vi "Plink Test.vi"() -> ()   [LabVIEW 2024]
panel:
  in  "format string":string="plink -pw changeme -batch -no-antispoof root@%s \"/opt/bin/maglab_rp_info\""
  in  "wait until completion? (T)":bool=TRUE
  in  "IP":string="192.168.1.120"
  in  "run minimized? (F)":bool
  out "return code":i32
  out "standard error":string
  out "standard output":string
  out "command":string
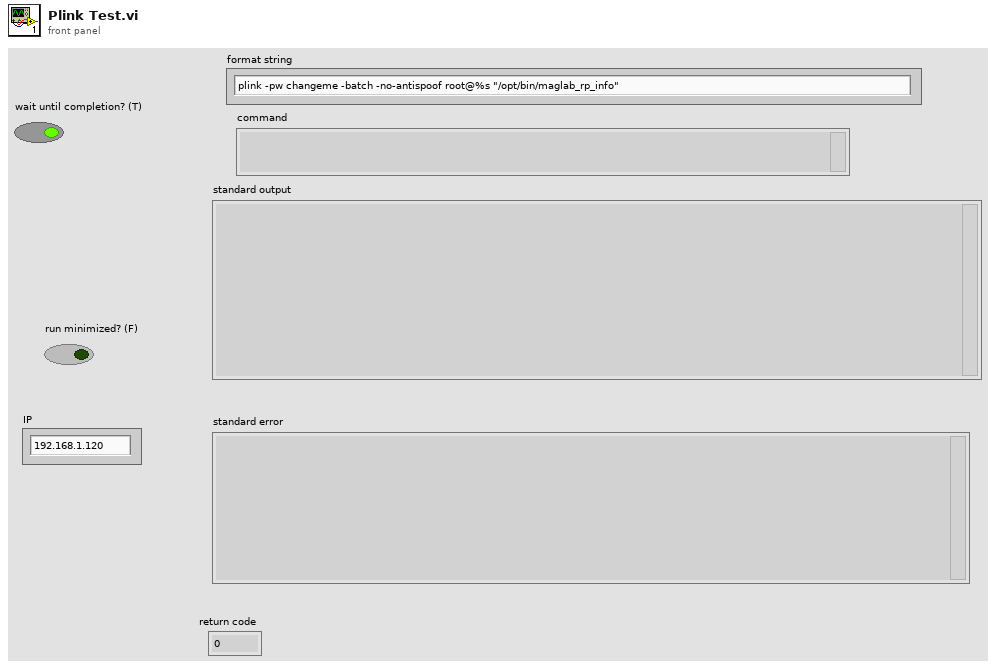
[diagram p1: front panel]
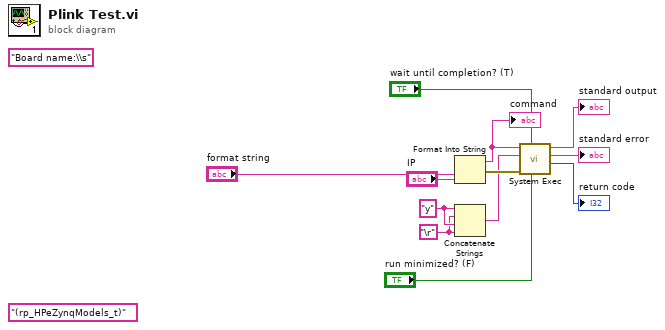
[diagram p0: block diagram]
diagram:
  w7 = "\r"
  w8 = "y" ("standard input")
  (unwired) "(rp_HPeZynqModels_t)"
  (unwired) "Board name:\\s"
  n1 = Format Into String(format string="format string", "IP") -> (resulting string=w9:string, error out=w11:errorcluster)  [unwired: 2 in]
  "command" <- w9
  n2 = Concatenate Strings(w8, w7, w8, w7) -> (w10:string)
  n3 = call <vilib>:"System Exec.vi"("run minimized? (F)"="run minimized? (F)", "wait until completion? (T)"="wait until completion? (T)", "error in (no error)"=w11, "standard input"=w10, "command line"=w9) -> ("return code"=→"return code":i32, "standard error"=→"standard error":string, "standard output"=→"standard output":string)  [unwired: 3 in, 1 out]
